vi "piezoDoubleWriteClose.vi"   [LabVIEW 2017]
uses:
  <vilib>/DAQmx/write.llb/DAQmx Write (Analog 1D DBL NChan 1Samp).vi
  globalDevices.vi
  <vilib>/DAQmx/miscellaneous.llb/DAQmx Fill In Error Info.vi
  <vilib>/DAQmx/create/channels.llb/DAQmx Create Channel (AO-Voltage-Basic).vi
  <vilib>/DAQmx/create/channels.llb/DAQmx Create Channel (AI-Voltage-Basic).vi
  <vilib>/DAQmx/read.llb/DAQmx Read (Analog DBL 1Chan 1Samp).vi
  Piezo/lvlib/Madlib.lvlib
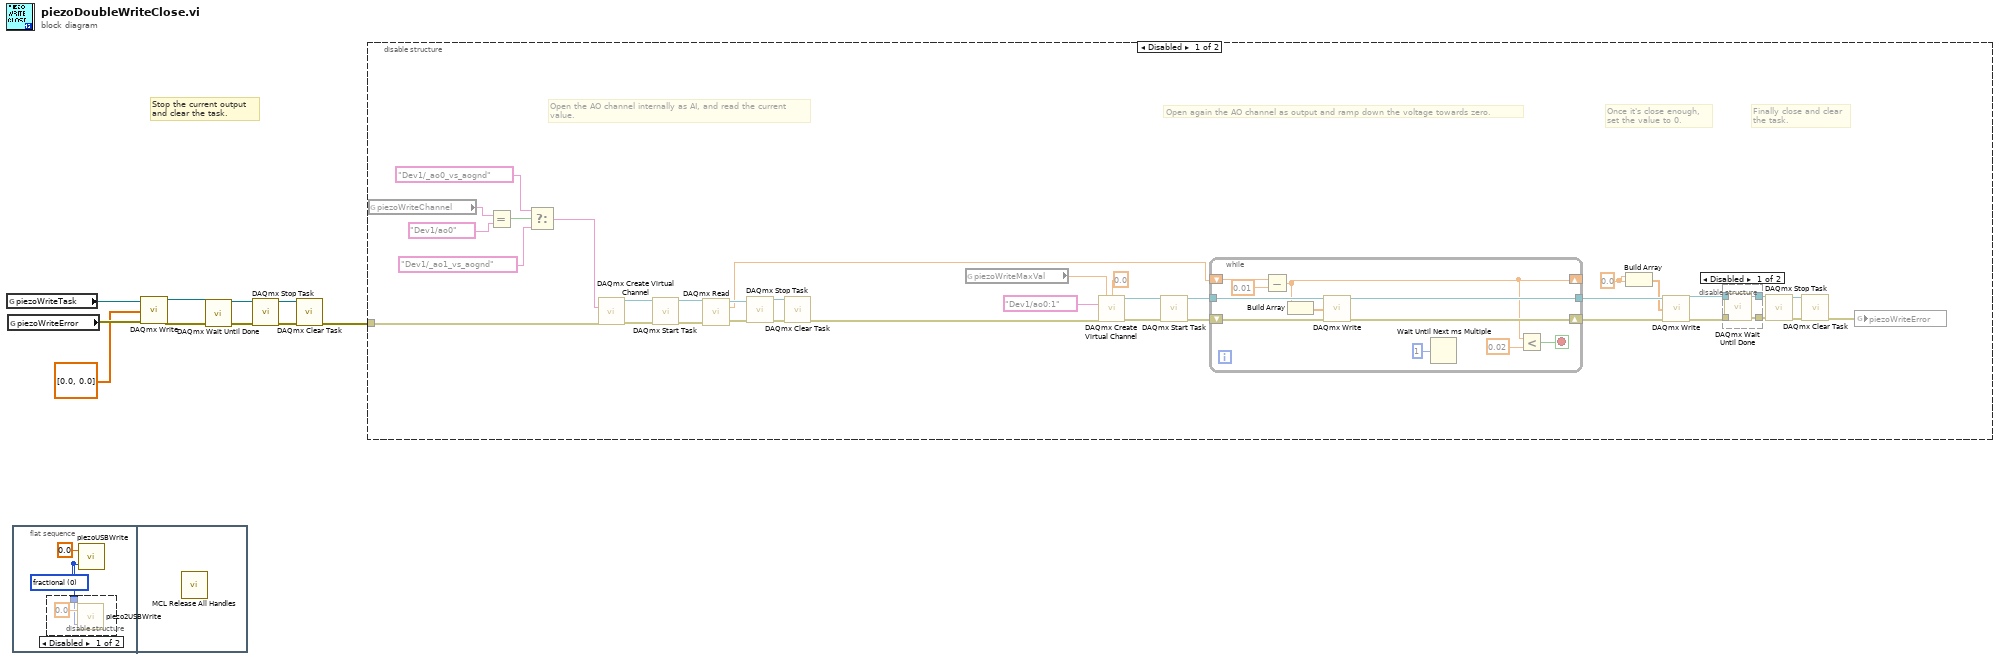
[diagram p0: block diagram]
diagram:
  # "Stop the current output\nand clear the task."
  n1 = global read "globalDevices.vi" "piezoWriteTask"() -> (w7:refnum<k21>)
  n2 = global read "globalDevices.vi" "piezoWriteError"() -> (w6:errorcluster)
  n3 = flat-sequence {
    frame #0 {
      w11 = u16 0 items=["fractional", "voltage (V)", "position (um)"] ("mode")
      n4 = disable-structure shown="Disabled" {
        disable-tunnel: w11 -> [w13 _]
        frame Disabled {
          n5 = call "piezo2USBWrite.vi"("mode"=w13, "position"=0.0) -> ()  [unwired: 1 in]
        }
        frame Enabled {
        }
      }
      n6 = call "piezoUSBWrite.vi"("mode"=w11, "position"=0.0) -> ()  [unwired: 1 in]
    }
    frame #1 {
      n7 = call "MCL Release All Handles.vi"() -> ()  [unwired: 12 in]
    }
  }
  n8 = call-poly <vilib>:"DAQmx Write.vi"("task/channels in"=w7, "data"=dbl[] [0.0, 0.0], "error in"=w6) -> ("task out"=w4:refnum<k21>, "error out"=w3:errorcluster)  [unwired: 10 in, 1 out]
  n9 = call <vilib>:"DAQmx Wait Until Done.vi"("task/channels in"=w4, "error in"=w3) -> ("task out"=w1:refnum<k21>, "error out"=w2:errorcluster)  [unwired: 12 in]
  n10 = call <vilib>:"DAQmx Stop Task.vi"("task/channels in"=w1, "error in"=w2) -> ("task out"=w9:refnum<k21>, "error out"=w10:errorcluster)  [unwired: 12 in]
  n11 = call <vilib>:"DAQmx Clear Task.vi"("task in"=w9, "error in"=w10) -> ("error out"=w8:errorcluster)  [unwired: 13 in]
  n12 = disable-structure shown="Disabled" {
    disable-tunnel: w8 -> [w30 _]
    frame Disabled {
      w21 = 0.0 ("data")
      # "Finally close and clear\nthe task."
      # "Once it's close enough,\nset the value to 0."
      # "Open again the AO channel as output and ramp down the voltage towards zero."
      # "Open the AO channel internally as AI, and read the current\nvalue."
      n13 = global read "globalDevices.vi" "piezoWriteChannel"() -> (w36:tag)
      n14 = Equal?(x=w36, y=tag "Dev1/ao0" ("physical channels")) -> (x = y?=w34:bool)
      n15 = Select(t=tag "Dev1/_ao0_vs_aognd" ("physical channels"), s=w34, f=tag "Dev1/_ao1_vs_aognd" ("physical channels")) -> (s? t:f=w31:tag)
      n16 = call-poly <vilib>:"DAQmx Create Virtual Channel.vi"("physical channels"=w31, "error in"=w30) -> ("task out"=w41:refnum<k21>, "error out"=w29:errorcluster)  [unwired: 12 in]
      n17 = call <vilib>:"DAQmx Start Task.vi"("task/channels in"=w41, "error in"=w29) -> ("task out"=w40:refnum<k21>, "error out"=w28:errorcluster)  [unwired: 12 in]
      n18 = call-poly <vilib>:"DAQmx Read.vi"("task/channels in"=w40, "error in"=w28) -> ("task out"=w39:refnum<k21>, "data"=w37:dbl, "error out"=w27:errorcluster)  [unwired: 11 in]
      n19 = call <vilib>:"DAQmx Stop Task.vi"("task/channels in"=w39, "error in"=w27) -> ("task out"=w43:refnum<k21>, "error out"=w42:errorcluster)  [unwired: 12 in]
      n20 = call <vilib>:"DAQmx Clear Task.vi"("task in"=w43, "error in"=w42) -> ("error out"=w38:errorcluster)  [unwired: 13 in]
      n21 = global read "globalDevices.vi" "piezoWriteMaxVal"() -> (w44:dbl)
      n22 = call-poly <vilib>:"DAQmx Create Virtual Channel.vi"("maximum value"=w44, "minimum value"=0.0, "physical channels"=tag "Dev1/ao0:1", "error in"=w38) -> ("task out"=w46:refnum<k21>, "error out"=w26:errorcluster)  [unwired: 10 in]
      n23 = call <vilib>:"DAQmx Start Task.vi"("task/channels in"=w46, "error in"=w26) -> ("task out"=w45:refnum<k21>, "error out"=w25:errorcluster)  [unwired: 12 in]
      n24 = while {
        shift-right: [w55] -> _
        shift-left: w37 -> [w64]
        tunnel: w45 -> [w60]
        tunnel: [w59] -> w24
        shift-right: [w56] -> w23
        shift-left: w25 -> [w57]
        stop <- w61 stop-if-true
        n25 = Subtract(x=w64, y=0.01) -> (x-y=w55:dbl)
        n26 = Build Array(w55, w55) -> (w54:dbl[])
        n27 = call-poly <vilib>:"DAQmx Write.vi"("task/channels in"=w60, "data"=w54, "error in"=w57) -> ("task out"=w59:refnum<k21>, "error out"=w56:errorcluster)  [unwired: 10 in, 1 out]
        n28 = Wait Until Next ms Multiple(millisecond multiple=u32 1) -> ()  [unwired: 1 out]
        n29 = Less?(x=w55, y=0.02) -> (x < y?=w61:bool)
      }
      n30 = Build Array(w21, w21) -> (w20:dbl[])
      n31 = call-poly <vilib>:"DAQmx Write.vi"("task/channels in"=w24, "data"=w20, "error in"=w23) -> ("task out"=w17:refnum<k21>, "error out"=w16:errorcluster)  [unwired: 10 in, 1 out]
      n32 = disable-structure shown="Disabled" {
        disable-tunnel: [w53 _] -> w19
        disable-tunnel: [w52 _] -> w18
        disable-tunnel: w17 -> [w51 _]
        disable-tunnel: w16 -> [w50 _]
        frame Disabled {
          n33 = call <vilib>:"DAQmx Wait Until Done.vi"("task/channels in"=w51, "error in"=w50) -> ("task out"=w53:refnum<k21>, "error out"=w52:errorcluster)  [unwired: 12 in]
        }
        frame Enabled {
        }
      }
      n34 = call <vilib>:"DAQmx Stop Task.vi"("task/channels in"=w19, "error in"=w18) -> ("task out"=w49:refnum<k21>, "error out"=w48:errorcluster)  [unwired: 12 in]
      n35 = call <vilib>:"DAQmx Clear Task.vi"("task in"=w49, "error in"=w48) -> ("error out"=w22:errorcluster)  [unwired: 13 in]
      n36 = global write "globalDevices.vi" "piezoWriteError"(w22) -> ()
    }
    frame Enabled {
    }
  }
